vi "Result.Parse Data File Name to SN, Time, Result_V2.vi"(11 "File Path":path) -> (1 "DateTime":timestamp, 2 "SN":string, 3 "Pass":bool)   [LabVIEW 2019]
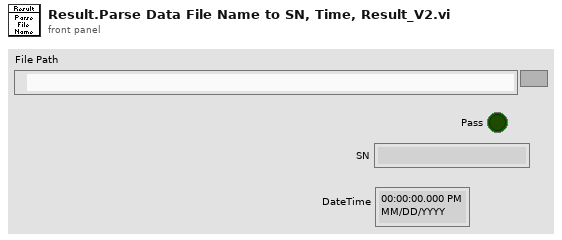
[diagram p1: front panel]
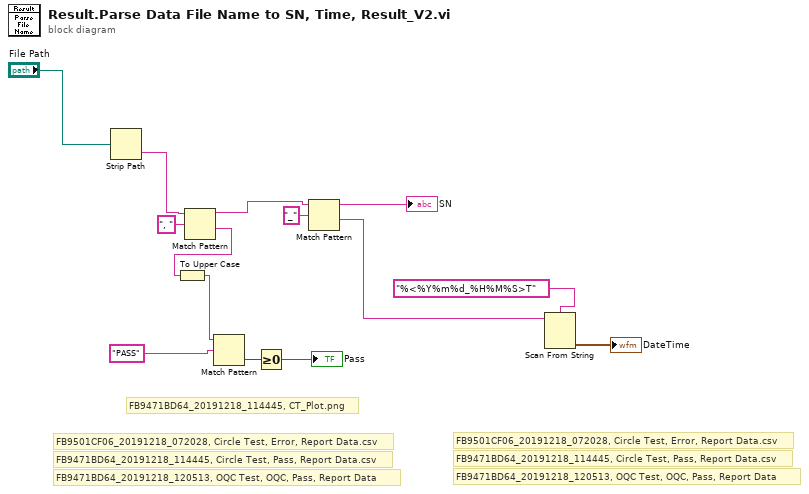
[diagram p0: block diagram]
diagram:
  # "FB9471BD64_20191218_120513, OQC Test, OQC, Pass, Report Data"
  # "FB9471BD64_20191218_114445, Circle Test, Pass, Report Data.csv"
  # "FB9501CF06_20191218_072028, Circle Test, Error, Report Data.csv"
  # "FB9471BD64_20191218_114445, CT_Plot.png"
  # "FB9471BD64_20191218_120513, OQC Test, OQC, Pass, Report Data"
  # "FB9471BD64_20191218_114445, Circle Test, Pass, Report Data.csv"
  # "FB9501CF06_20191218_072028, Circle Test, Error, Report Data.csv"
  n1 = Strip Path(path="File Path") -> (name=w12:string)  [unwired: 1 out]
  n2 = Match Pattern(string=w12, regular expression=", ") -> (before substring=w5:string, after substring=w11:string)  [unwired: 1 in, 2 out]
  n3 = To Upper Case(1:w11) -> (0:w10:string)
  n4 = Match Pattern(string=w10, regular expression="PASS") -> (offset past match=w8:i32)  [unwired: 1 in, 3 out]
  n5 = Greater Or Equal To 0?(x=w8) -> (x >= 0?=→"Pass":bool)
  n6 = Match Pattern(string=w5, regular expression="_") -> (before substring=→"SN":string, after substring=w2:string)  [unwired: 1 in, 2 out]
  n7 = Scan From String(format string="%<%Y%m%d_%H%M%S>T", input string=w2) -> (output 1=→"DateTime":timestamp)  [unwired: 3 in, 3 out]
